vi "Read Gain.vi"(8 "error in (no error)":errorcluster, 11 "SOL Camera in":refnum<class "PL SOL Instruments Camera.lvclass">) -> (0 "error out":errorcluster, 2 "gain":dbl, 3 "SOL Camera out":refnum<class "PL SOL Instruments Camera.lvclass">)   [LabVIEW 2015, in "PL SOL Instruments Camera.lvclass"]
doc: "Reads gain."
uses:
  PL SOL Instruments Camera.lvclass
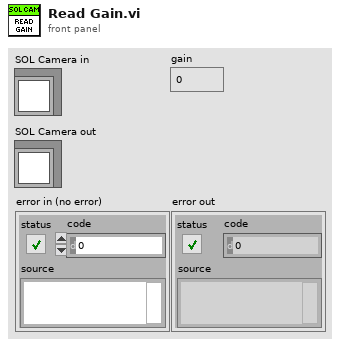
[diagram p1: front panel]
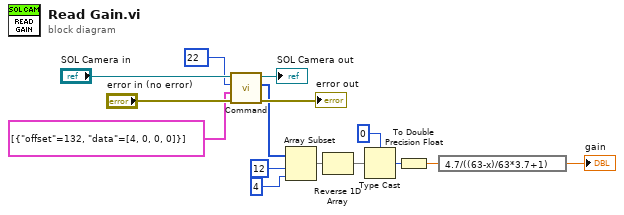
[diagram p0: block diagram]
diagram:
  n1 = call "Command.vi"("error in (no error)"="error in (no error)", "data"=cluster{"offset":u32, "data":u8[]}[] [{"offset"=132, "data"=[4, 0, 0, 0]}], "command"=u8 22, "SOL Camera in"="SOL Camera in") -> ("error out"=→"error out":errorcluster, "response"=w1:u8[], "SOL Camera out"=→"SOL Camera out":refnum<class "PL SOL Instruments Camera.lvclass">)  [unwired: 5 in]
  n2 = Array Subset(array=w1, index=12, length=4) -> (w9:u8[])
  n3 = Reverse 1D Array(array=w9) -> (reversed array=w7:u8[])
  n4 = Type Cast(type=u32 0, x=w7) -> (*(type *) &x=w6:u32)
  n5 = To Double Precision Float(number=w6) -> (double precision float=w5:dbl)
  n6 = expression code="4.7/((63-x)/63*3.7+1)"(w5) -> (→"gain":dbl)
